vi "Q-Remove.vi"(7 "Queue Type":T1, 8 "error in":errorcluster, 9 "timeout in ms (-1)":i32=-1, 11 "Q Name":string) -> (0 "error out":errorcluster, 1 "Index":i32, 2 "Analog Data":waveform(dbl)[](array[waveform]), 3 "Digital Data":digitalwaveform[](array[waveform]), 4 "timed out?":bool, 5 "Variant Data":variant[](array[variant]))   [LabVIEW 2016]
uses:
  PSDAQEG_Task Queue Type.ctl
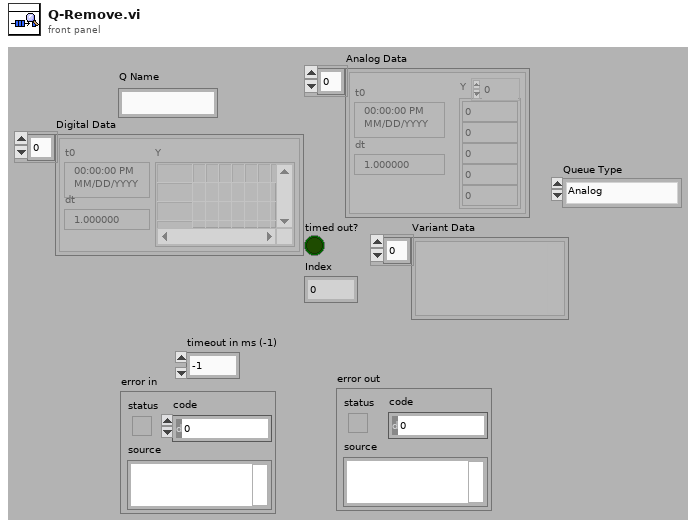
[diagram p1: front panel]
types:
  T1 = typedef "PSDAQEG_Task Queue Type.ctl" = enum16{"Analog", "Digital", "Variant"}
  T2 = cluster{"max queue size (-1, unlimited)":i32, "Waveform":waveform(dbl)[]}
  T3 = cluster{"max queue size (-1, unlimited)":i32, digitalwaveform[]}
  T4 = cluster{"max queue size (-1, unlimited)":i32, variant[]}
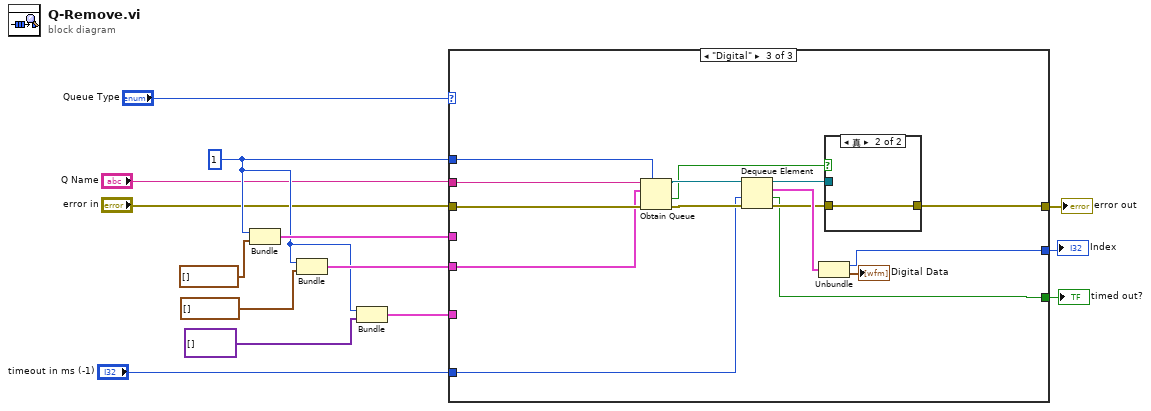
[diagram p0: block diagram]
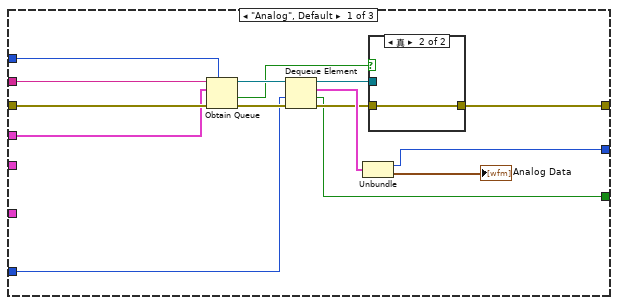
[diagram p2: hidden frame]
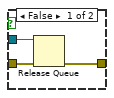
[diagram p3: hidden frame]
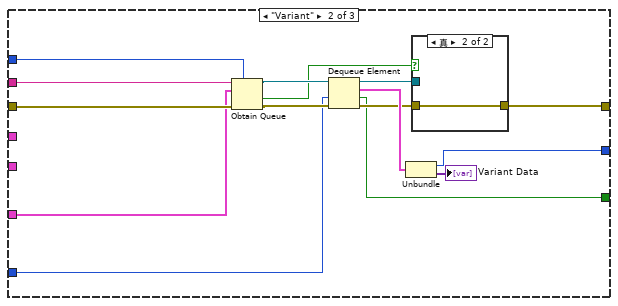
[diagram p4: hidden frame]
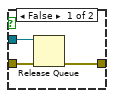
[diagram p5: hidden frame]
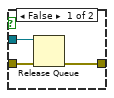
[diagram p6: hidden frame]
diagram:
  w8 = 1 ("max queue size (-1, unlimited)")
  n1 = Bundle("max queue size (-1, unlimited)"=w8, "Waveform"=waveform(dbl)[] []) -> (w10:T2)  [unwired: 1 in]
  n2 = Bundle("max queue size (-1, unlimited)"=w8, digitalwaveform[] []) -> (w11:T3)  [unwired: 1 in]
  n3 = Bundle("max queue size (-1, unlimited)"=w8, variant[] []) -> (w7:T4)  [unwired: 1 in]
  n4 = case shown="\"Digital\"" "Queue Type" {
    tunnel: "Q Name" -> [w28 w47 w67]
    tunnel: "error in" -> [w29 w48 w66]
    tunnel: w8 -> [w27 w46 w65]
    tunnel: w11 -> [_ _ w64]
    tunnel: [w17 w35 w55] -> w3
    tunnel: w10 -> [w26 _ _]
    tunnel: w7 -> [_ w45 _]
    tunnel: "timeout in ms (-1)" -> [w15 w39 w58]
    tunnel: [w18 w36 w56] -> w2
    tunnel: [w16 w37 w57] -> w1
    frame "Analog", Default {
      n5 = Obtain Queue(max queue size (-1, unlimited)=w27, name (unnamed)=w28, element data type=w26, error in (no error)=w29) -> (queue out=w22:refnum<queue>, created new?=w20:bool, error out=w21:errorcluster)  [unwired: 1 in]
      n6 = Dequeue Element(queue=w22, timeout in ms (-1)=w15, error in (no error)=w21) -> (queue out=w23:refnum<queue>, element=w25:T2, timed out?=w16:bool, error out=w24:errorcluster)
      n7 = Unbundle(w25) -> ("max queue size (-1, unlimited)"=w18:i32, "Waveform"=→"Analog Data":waveform(dbl)[])
      n8 = case shown="真" w20 {
        tunnel: w23 -> [w32 _]
        tunnel: w24 -> [w31 w33]
        tunnel: [w30 w33] -> w17
        frame False {
          n9 = Release Queue(queue=w32, error in (no error)=w31) -> (error out=w30:errorcluster)  [unwired: 1 in, 2 out]
        }
        frame True {
        }
      }
    }
    frame "Variant" {
      n10 = Obtain Queue(max queue size (-1, unlimited)=w46, name (unnamed)=w47, element data type=w45, error in (no error)=w48) -> (queue out=w40:refnum<queue>, created new?=w38:bool, error out=w41:errorcluster)  [unwired: 1 in]
      n11 = Dequeue Element(queue=w40, timeout in ms (-1)=w39, error in (no error)=w41) -> (queue out=w42:refnum<queue>, element=w44:T4, timed out?=w37:bool, error out=w43:errorcluster)
      n12 = Unbundle(w44) -> ("max queue size (-1, unlimited)"=w36:i32, →"Variant Data":variant[])
      n13 = case shown="真" w38 {
        tunnel: w42 -> [w51 _]
        tunnel: w43 -> [w50 w52]
        tunnel: [w49 w52] -> w35
        frame False {
          n14 = Release Queue(queue=w51, error in (no error)=w50) -> (error out=w49:errorcluster)  [unwired: 1 in, 2 out]
        }
        frame True {
        }
      }
    }
    frame "Digital" {
      n15 = Obtain Queue(max queue size (-1, unlimited)=w65, name (unnamed)=w67, element data type=w64, error in (no error)=w66) -> (queue out=w60:refnum<queue>, created new?=w54:bool, error out=w59:errorcluster)  [unwired: 1 in]
      n16 = Dequeue Element(queue=w60, timeout in ms (-1)=w58, error in (no error)=w59) -> (queue out=w61:refnum<queue>, element=w63:T3, timed out?=w57:bool, error out=w62:errorcluster)
      n17 = Unbundle(w63) -> ("max queue size (-1, unlimited)"=w56:i32, →"Digital Data":digitalwaveform[])
      n18 = case shown="真" w54 {
        tunnel: w61 -> [w70 _]
        tunnel: w62 -> [w69 w71]
        tunnel: [w68 w71] -> w55
        frame False {
          n19 = Release Queue(queue=w70, error in (no error)=w69) -> (error out=w68:errorcluster)  [unwired: 1 in, 2 out]
        }
        frame True {
        }
      }
    }
  }
  "error out" <- w3
  "timed out?" <- w1
  "Index" <- w2
